vi "testErrorPropagation.vi"(8 "error in (no error)":errorcluster, 11 "TestCase in":refnum<class "EasyXMLTest.lvclass">) -> (0 "error out":errorcluster, 3 "TestCase out":refnum<class "EasyXMLTest.lvclass">)   [LabVIEW 2011, in "EasyXMLTest.lvclass"]
doc: "Verify that error in is not overwritten"
uses:
  EasyXMLTest.lvclass
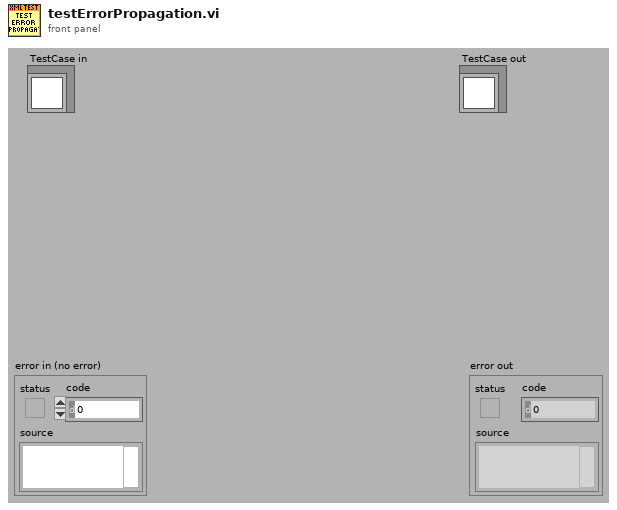
[diagram p1: front panel]
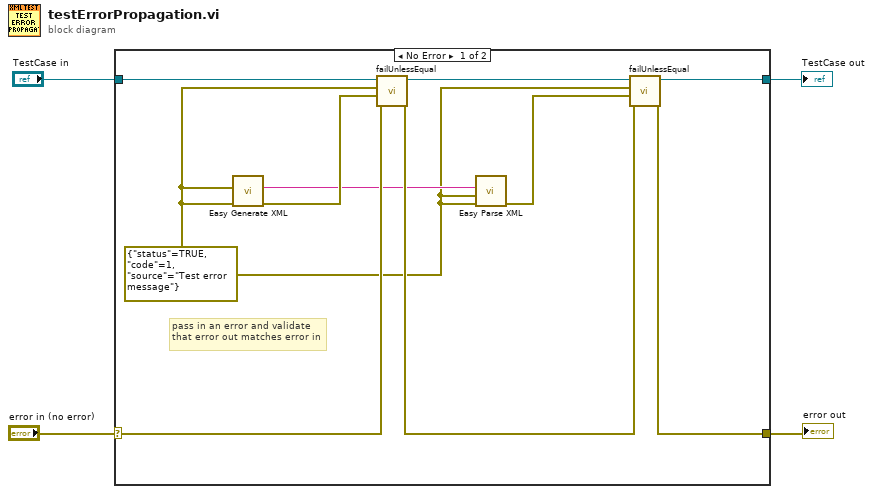
[diagram p0: block diagram]
diagram:
  n1 = case shown="No Error" "error in (no error)" {
    selector: "error in (no error)" -> [w13 w16]
    tunnel: [w9 w16] -> w3
    tunnel: [w11 w15] -> w1
    tunnel: "TestCase in" -> [w14 w15]
    frame No Error {
      w5 = errorcluster {"status"=TRUE, "code"=1, "source"="Test error message"} ("error IO")
      # "pass in an error and validate that error out matches error in"
      n2 = call "Easy Generate XML.vi"("error in (no error)"=w5, "LabVIEW Data"=w5) -> ("error out"=w8:errorcluster, "XML String"=w7:string)  [unwired: 8 in]
      n3 = call-dynamic "failUnlessEqual.vi"("error in (no error)"=w13, "y"=w8, "x"=w5, "TestCase in"=w14) -> ("error out"=w10:errorcluster, "TestCase out"=w12:refnum<class "EasyXMLTest.lvclass">)  [unwired: 6 in]
      n4 = call "Easy Parse XML.vi"("error in (no error)"=w5, "LabVIEW Data (Type)"=w5, "XML String"=w7) -> ("error out"=w6:errorcluster)  [unwired: 7 in, 1 out]
      n5 = call-dynamic "failUnlessEqual.vi"("error in (no error)"=w10, "y"=w6, "x"=w5, "TestCase in"=w12) -> ("error out"=w9:errorcluster, "TestCase out"=w11:refnum<class "EasyXMLTest.lvclass">)  [unwired: 6 in]
    }
    frame Error {
    }
  }
  "error out" <- w3
  "TestCase out" <- w1
